vi "stage_move_absolute.vi"(7 "Stage Name":string, 8 "error in (no error)":errorcluster, 9 "wait_for_done":bool, 10 "Position":dbl, 11 "galvo in":refnum<class "galvo.lvclass">) -> (0 "error out":errorcluster, 3 "galvo out":refnum<class "galvo.lvclass">)   [LabVIEW 2015, in "galvo.lvclass"]
uses:
  galvo.lvclass
  galvo.lvclass/galvo.ctl
  <vilib>/DAQmx/write.llb/DAQmx Write (Analog DBL 1Chan 1Samp).vi
  <vilib>/DAQmx/miscellaneous.llb/DAQmx Fill In Error Info.vi
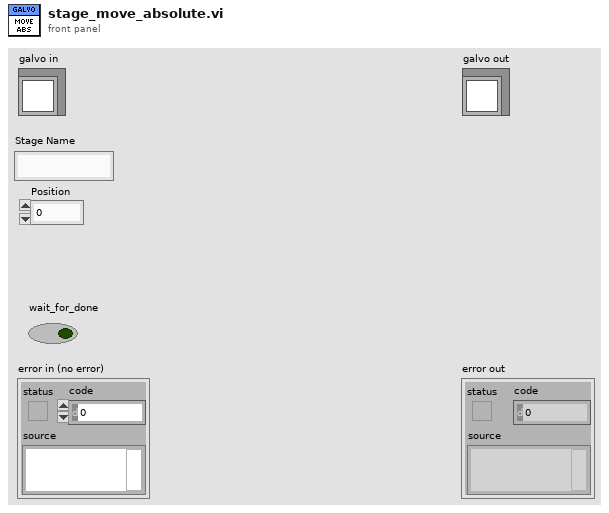
[diagram p1: front panel]
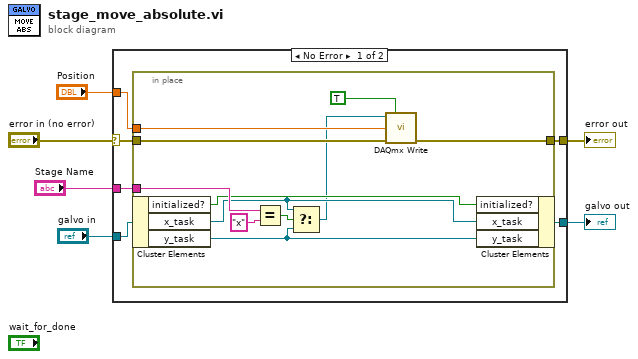
[diagram p0: block diagram]
diagram:
  n1 = case shown="No Error" "error in (no error)" {
    selector: "error in (no error)" -> [w8 w24]
    tunnel: "galvo in" -> [w12 w25]
    tunnel: "Stage Name" -> [w11 _]
    tunnel: "Position" -> [w10 _]
    tunnel: [w9 w25] -> w2
    tunnel: [w7 w24] -> w1
    frame No Error {
      n2 = in-place {
        in-place-border: w11 -> [w22]
        in-place-border: w10 -> [w20]
        in-place-border: w8 -> [w17]
        in-place-border: [w16] -> w7
        n3 = in-place-cluster #1(w12) -> ("initialized?"=w15:bool, "x_task"=w19:refnum<k21>, "y_task"=w18:refnum<k21>)
        n4 = Equal?(x=w22, y="x") -> (x = y?=w21:bool)
        n5 = Select(t=w19, s=w21, f=w18) -> (s? t:f=w13:refnum<k21>)
        n6 = call-poly <vilib>:"DAQmx Write.vi"("task/channels in"=w13, "auto start"=TRUE, "data"=w20, "error in"=w17) -> ("error out"=w16:errorcluster)  [unwired: 9 in, 2 out]
        n7 = in-place-cluster #1("initialized?"=w15, "x_task"=w19, "y_task"=w18) -> (w9:refnum<class "galvo.lvclass">)
      }
    }
    frame Error {
    }
  }
  "error out" <- w1
  "galvo out" <- w2
